vi "Serial.vi"(8 "error in (no error)":errorcluster, 9 "Clear Log":bool, 10 "write buffer":string="UA[3]\r\n", 11 "VISA resource name":refnum<visa-resource-name>="COM6") -> (0 "error out":errorcluster, 2 "read buffer":string)   [LabVIEW 2017]
uses:
  <vilib>/Instr/_visa.llb/VISA Configure Serial Port (Instr).vi
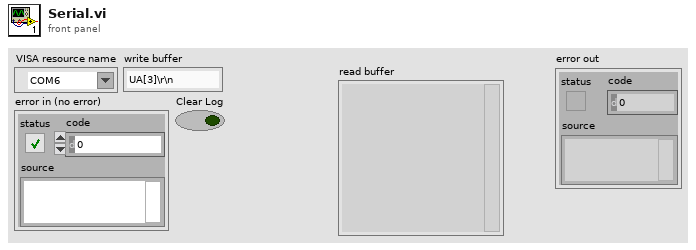
[diagram p1: front panel]
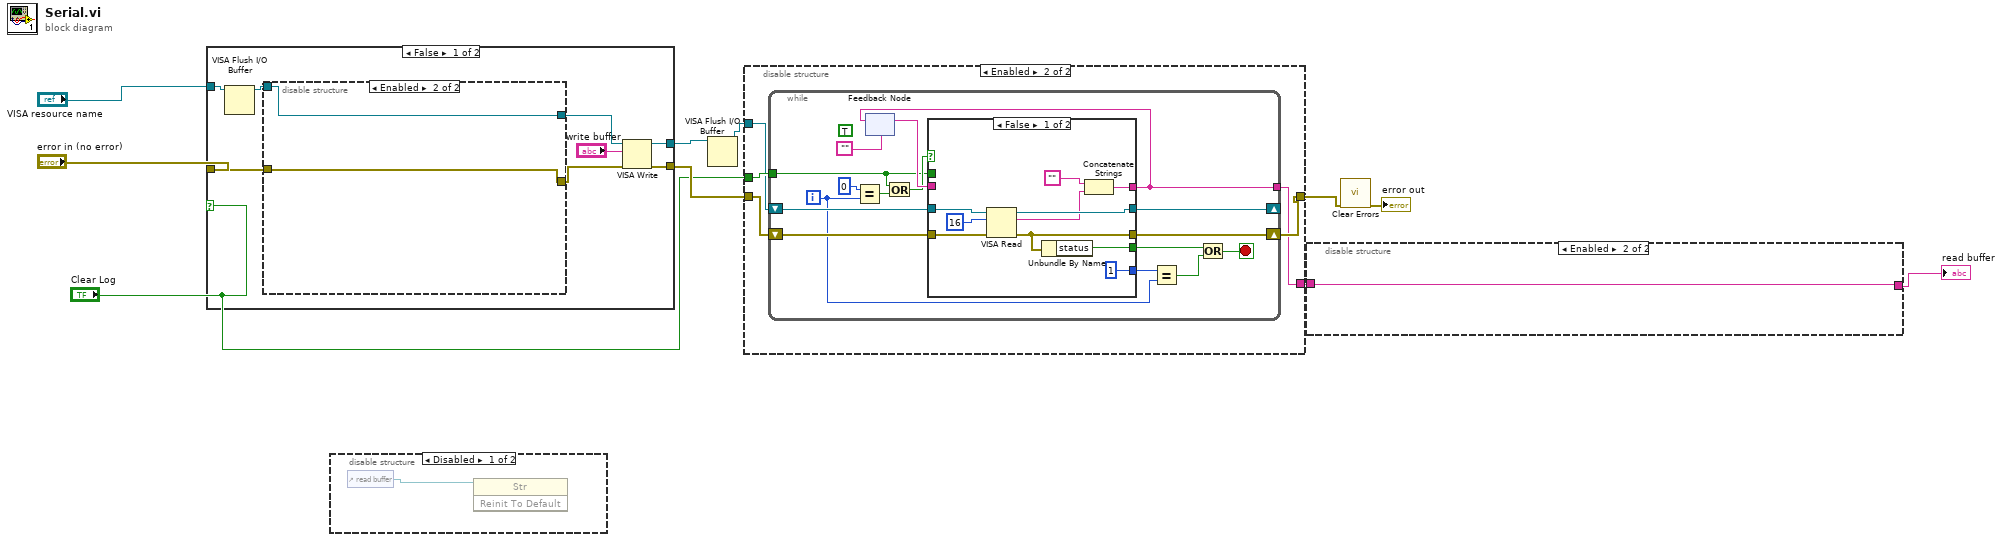
[diagram p0: block diagram]
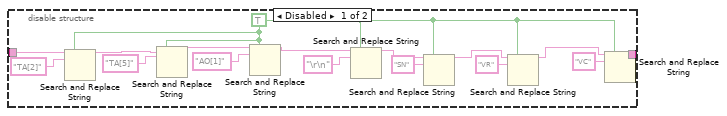
[diagram p2: hidden frame]
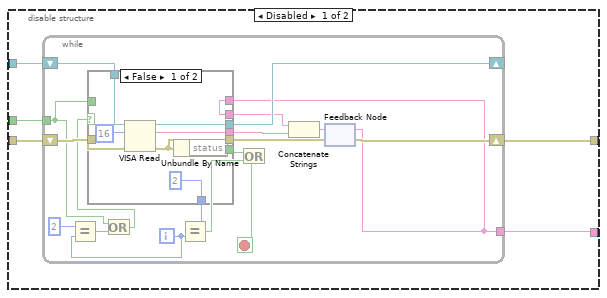
[diagram p3: hidden frame]
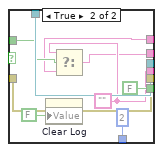
[diagram p4: hidden frame]
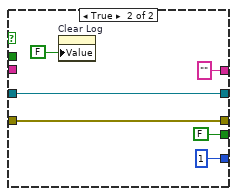
[diagram p5: hidden frame]
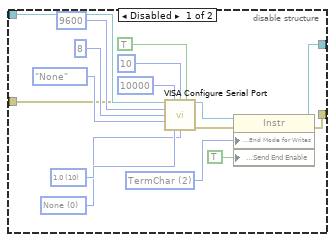
[diagram p7: hidden frame]
diagram:
  n1 = case shown="False" "Clear Log" {
    tunnel: "VISA resource name" -> [w13 w38]
    tunnel: "error in (no error)" -> [w12 w37]
    tunnel: [w16 w38] -> w2
    tunnel: [w15 w37] -> w6
    frame False {
      n2 = VISA Flush I/O Buffer(VISA resource name=w13) -> (VISA resource name out=w11:refnum<visa-resource-name>)  [unwired: 2 in, 1 out]
      n3 = disable-structure shown="Enabled" {
        disable-tunnel: w11 -> [w34 w36]
        disable-tunnel: w12 -> [w28 w35]
        disable-tunnel: [w23 w36] -> w17
        disable-tunnel: [w22 w35] -> w18
        frame Disabled {
          w20 = u16 2 items=["None", "LastBit", "TermChar", "Break"] ("Serial Settings:Serial End Mode for Writes")
          w26 = u16 0 items=["None", "XON/XOFF", "RTS/CTS", "XON/XOFF & RTS/CTS", "DTR/DSR", "XON/XOFF & DTR/DSR"] ("flow control (0:none)")
          w27 = u16 10 items=["1.0"=10, "1.5"=15, "2.0"=20] ("stop bits (10: 1 bit)")
          n4 = call-poly "VISA Configure Serial Port"("VISA resource name"=w34, "timeout (10sec)"=u32 10000, "termination char\n(0xA = '\\n' = LF)"=u8 10 ("termination char\n(0xA = '\\n' = LF)"), "Enable Termination\nChar (T)"=TRUE ("Enable Termination\nChar (T)"), "baud rate (9600)"=u32 9600, "data bits (8)"=u16 8, "parity (0:none)"=enum16{"None", "Odd", "Even", "Mark", "Space"}."None", "error in (no error)"=w28, "stop bits (10: 1 bit)"=w27, "flow control (0:none)"=w26) -> ("VISA resource name out"=w24:refnum<visa-resource-name>, "error out"=w25:errorcluster)  [unwired: 4 in]
          n5 = property class="Instr"(reference=w24, error in=w25, "Serial Settings:End Mode for Writes"=w20, "Message Based Settings:Send End Enable"=TRUE) -> (reference out=w23:refnum<visa-resource-name>, error out=w22:errorcluster)
        }
        frame Enabled {
        }
      }
      n6 = VISA Write(VISA resource name=w17, write buffer="write buffer", error in (no error)=w18) -> (VISA resource name out=w16:refnum<visa-resource-name>, error out=w15:errorcluster)  [unwired: 1 out]
    }
    frame True {
    }
  }
  n7 = disable-structure shown="Disabled" {
    frame Disabled {
      n8 = control-ref of="read buffer"() -> (w39:refnum<vi>)
      n9 = invoke class="Str" method="Reinit To Default"(reference=w39) -> ()  [unwired: 2 in, 3 out]
    }
    frame Enabled {
    }
  }
  n10 = VISA Flush I/O Buffer(VISA resource name=w2) -> (VISA resource name out=w1:refnum<visa-resource-name>)  [unwired: 2 in, 1 out]
  n11 = disable-structure shown="Enabled" {
    disable-tunnel: [w44 w81] -> w9
    disable-tunnel: w1 -> [w43 w83]
    disable-tunnel: w6 -> [w42 w82]
    disable-tunnel: "Clear Log" -> [w41 w84]
    disable-tunnel: [w40 w80] -> w4
    frame Disabled {
      n12 = while {
        shift-right: [w61] -> _
        shift-left: w43 -> [w55]
        shift-right: [w59] -> w44
        shift-left: w42 -> [w54]
        tunnel: [w52] -> w40
        tunnel: w41 -> [w45]
        i -> [w49]
        stop <- w57 stop-if-true
        n13 = Equal?(x=2, y=w49) -> (x = y?=w47:bool)
        n14 = Or(x=w45, y=w47) -> (x .or. y?=w46:bool)
        n15 = feedback #1() -> (w52:string)  [unwired: 1 in]
        n16 = case shown="False" w46 {
          tunnel: [w70 w79] -> w61
          tunnel: [w69 w73] -> w60
          tunnel: [w67 w78] -> w59
          tunnel: [w66 FALSE ("status")] -> w56
          tunnel: w55 -> [w65 w79]
          tunnel: w54 -> [w64 w78]
          tunnel: w52 -> [w63 w72]
          tunnel: [w63 w71] -> w51
          tunnel: [2 ("x") 2 ("x")] -> w50
          tunnel: w45 -> [_ w74]
          frame False {
            n17 = VISA Read(VISA resource name=w65, byte count=u32 16, error in (no error)=w64) -> (VISA resource name out=w70:refnum<visa-resource-name>, read buffer=w69:string, error out=w67:errorcluster)  [unwired: 1 out]
            n18 = Unbundle By Name(w67) -> ("status"=w66:bool)
          }
          frame True {
            w73 = ""
            n19 = property on="Clear Log" class="Bool (strict)"("Value"=FALSE ("Clear Log")) -> ()  [unwired: 2 in, 2 out]
            n20 = Select(t=w73, s=w74, f=w72) -> (s? t:f=w71:string)
          }
        }
        n21 = Equal?(x=w50, y=w49) -> (x = y?=w58:bool)
        n22 = Or(x=w56, y=w58) -> (x .or. y?=w57:bool)
        n23 = Concatenate Strings(w51, w60) -> (w53:string)
        n24 = feedback-in #1(w53) -> ()
      }
    }
    frame Enabled {
      n25 = while {
        shift-right: [w100] -> _
        shift-left: w83 -> [w97]
        shift-right: [w99] -> w81
        shift-left: w82 -> [w96]
        tunnel: w84 -> [w89]
        tunnel: [w85] -> w80
        i -> [w93]
        stop <- w86 stop-if-true
        (unwired) TRUE
        n26 = Equal?(x=0, y=w93) -> (x = y?=w91:bool)
        n27 = feedback #2("") -> (w95:string)
        n28 = Or(x=w89, y=w91) -> (x .or. y?=w90:bool)
        n29 = case shown="False" w90 {
          tunnel: [w110 w116] -> w100
          tunnel: [w108 w115] -> w99
          tunnel: [w107 FALSE ("status")] -> w98
          tunnel: w97 -> [w106 w116]
          tunnel: w96 -> [w105 w115]
          tunnel: w95 -> [_ _]
          tunnel: [1 ("x") 1 ("x")] -> w94
          tunnel: w89 -> [_ _]
          tunnel: [w103 ""] -> w85
          frame False {
            n30 = VISA Read(VISA resource name=w106, byte count=u32 16, error in (no error)=w105) -> (VISA resource name out=w110:refnum<visa-resource-name>, read buffer=w101:string, error out=w108:errorcluster)  [unwired: 1 out]
            n31 = Unbundle By Name(w108) -> ("status"=w107:bool)
            n32 = Concatenate Strings("", w101) -> (w103:string)
          }
          frame True {
            n33 = property on="Clear Log" class="Bool (strict)"("Value"=FALSE ("Clear Log")) -> ()  [unwired: 2 in, 2 out]
          }
        }
        n34 = feedback-in #2(w85) -> ()
        n35 = Equal?(x=w94, y=w93) -> (x = y?=w87:bool)
        n36 = Or(x=w98, y=w87) -> (x .or. y?=w86:bool)
      }
    }
  }
  n37 = disable-structure shown="Enabled" {
    disable-tunnel: w4 -> [w123 w133]
    disable-tunnel: [w118 w133] -> w3
    frame Disabled {
      w117 = TRUE ("replace all? (F)")
      n38 = Search and Replace String(replace all?=w117, input string=w123, search string="TA[2]" ("substring (\"\")")) -> (result string=w124:string)  [unwired: 5 in, 3 out]
      n39 = Search and Replace String(replace all?=w117, input string=w124, search string="TA[5]" ("substring (\"\")")) -> (result string=w130:string)  [unwired: 5 in, 3 out]
      n40 = Search and Replace String(replace all?=w117, input string=w130, search string="AO[1]" ("substring (\"\")")) -> (result string=w128:string)  [unwired: 5 in, 3 out]
      n41 = Search and Replace String(replace all?=w117, input string=w128, search string="\r\n" ("substring (\"\")")) -> (result string=w127:string)  [unwired: 5 in, 3 out]
      n42 = Search and Replace String(replace all?=w117, input string=w127, search string="SN") -> (result string=w121:string)  [unwired: 5 in, 3 out]
      n43 = Search and Replace String(replace all?=w117, input string=w121, search string="VR") -> (result string=w119:string)  [unwired: 5 in, 3 out]
      n44 = Search and Replace String(replace all?=w117, input string=w119, search string="VC") -> (result string=w118:string)  [unwired: 5 in, 3 out]
    }
    frame Enabled {
    }
  }
  "read buffer" <- w3
  n45 = call <vilib>:"Clear Errors.vi"("error in (no error)"=w9) -> ("error out"=→"error out":errorcluster)  [unwired: 5 in, 1 out]
